vi "GetStructures.vi"(6 "error in":errorcluster, 9 "VI Interpreter in":refnum<class "VI Interpreter.lvclass">) -> (0 "error out":errorcluster, 3 "VI Interpreter out":refnum<class "VI Interpreter.lvclass">)   [LabVIEW 2014, in "VI Interpreter.lvclass"]
uses:
  VI Interpreter.lvclass
  Diagram/Diagram.lvclass/Diagram.ctl
  Structure/Structure.lvclass/Structure.ctl
  Structure/Structure.lvclass
  Diagram/Diagram.lvclass
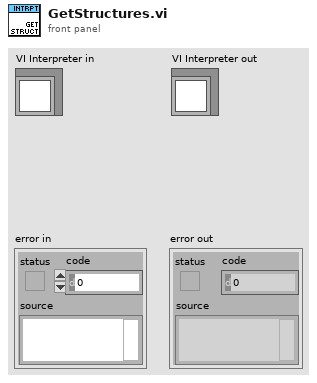
[diagram p1: front panel]
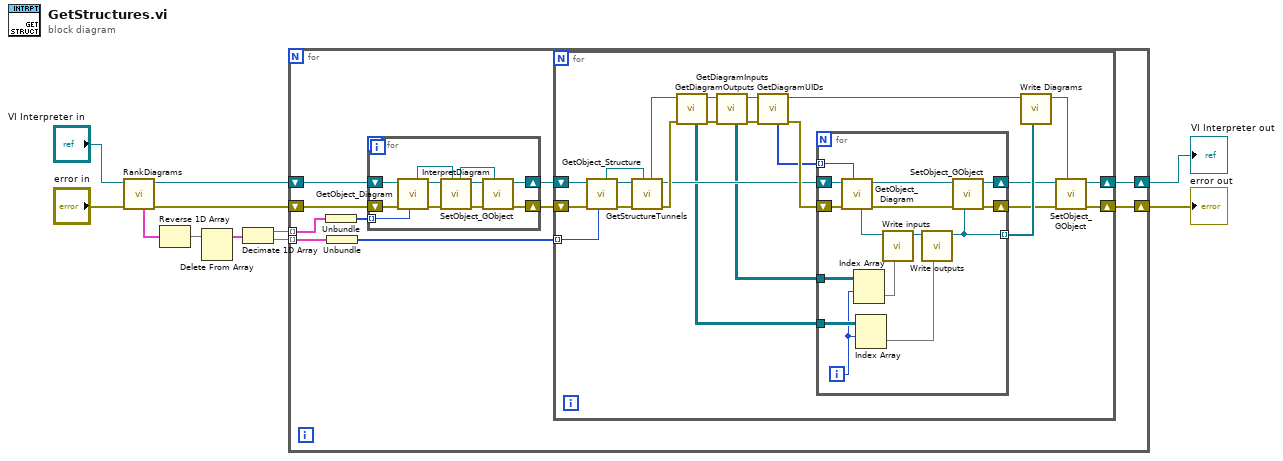
[diagram p0: block diagram]
diagram:
  n1 = call "RankDiagrams.vi"("error in"="error in", "VI Interpreter in"="VI Interpreter in") -> ("error out"=w3:errorcluster, "VI Interpreter out"=w4:refnum<class "VI Interpreter.lvclass">, "Rank"=w9:cluster{"nodes":i32[]}[])  [unwired: 5 in]
  n2 = Reverse 1D Array(array=w9) -> (reversed array=w8:cluster{"nodes":i32[]}[])
  n3 = Delete From Array(array=w8) -> (array with subset deleted=w7:cluster{"nodes":i32[]}[])  [unwired: 2 in, 1 out]
  n4 = Decimate 1D Array(w7) -> (w6:cluster{"nodes":i32[]}[], w5:cluster{"nodes":i32[]}[])
  n5 = for {
    tunnel: w6 -> [w13] mode=indexing
    tunnel: w5 -> [w21] mode=indexing
    shift-right: [w19] -> w1
    shift-left: w4 -> [w15]
    shift-right: [w18] -> w2
    shift-left: w3 -> [w17]
    n6 = Unbundle(w13) -> ("nodes"=w12:i32[])
    n7 = Unbundle(w21) -> ("nodes"=w20:i32[])
    n8 = for {
      shift-right: [w25] -> w16
      shift-left: w17 -> [w32]
      shift-right: [w26] -> w14
      shift-left: w15 -> [w31]
      tunnel: w12 -> [w22] mode=indexing
      n9 = call "GetObject_Diagram.vi"("UID"=w22, "error in"=w32, "VI Interpreter in"=w31) -> ("error out"=w29:errorcluster, "VI Interpreter out"=w30:refnum<class "VI Interpreter.lvclass">, "Diagram"=w23:refnum<class "Diagram.lvclass">)  [unwired: 3 in, 1 out]
      n10 = call "InterpretDiagram.vi"("Diagram"=w23, "error in"=w29, "VI Interpreter in"=w30) -> ("error out"=w27:errorcluster, "VI Interpreter out"=w28:refnum<class "VI Interpreter.lvclass">, "Diagram out"=w24:refnum<class "Diagram.lvclass">)  [unwired: 4 in]
      n11 = call "SetObject_GObject.vi"("GObject"=w24, "error in"=w27, "VI Interpreter in"=w28) -> ("error out"=w25:errorcluster, "VI Interpreter out"=w26:refnum<class "VI Interpreter.lvclass">)  [unwired: 5 in]
    }
    n12 = for {
      shift-right: [w35] -> w19
      shift-left: w14 -> [w56]
      tunnel: w20 -> [w54] mode=indexing
      shift-right: [w34] -> w18
      shift-left: w16 -> [w55]
      n13 = call "GetObject_Structure.vi"("UID"=w54, "error in"=w55, "VI Interpreter in"=w56) -> ("error out"=w51:errorcluster, "VI Interpreter out"=w53:refnum<class "VI Interpreter.lvclass">, "structure"=w52:refnum<class "Structure.lvclass">)  [unwired: 3 in, 1 out]
      n14 = call "GetStructureTunnels.vi"("Structure in"=w52, "error in"=w51, "VI Interpreter in"=w53) -> ("error out"=w45:errorcluster, "VI Interpreter out"=w43:refnum<class "VI Interpreter.lvclass">, "Structure out"=w48:refnum<class "Structure.lvclass">)  [unwired: 4 in]
      n15 = call-dynamic "GetDiagramOutputs.vi"("error in"=w45, "Structure in"=w48) -> ("error out"=w47:errorcluster, "Structure out"=w50:refnum<class "Structure.lvclass">, "output terminals"=w40:refnum<class "Terminal.lvclass">[][])  [unwired: 5 in]
      n16 = call-dynamic "GetDiagramInputs.vi"("error in"=w47, "Structure in"=w50) -> ("error out"=w46:errorcluster, "Structure out"=w49:refnum<class "Structure.lvclass">, "inputs terminals"=w41:refnum<class "Terminal.lvclass">[][])  [unwired: 5 in]
      n17 = call-dynamic "GetDiagramUIDs.vi"("error in"=w46, "Structure in"=w49) -> ("error out"=w44:errorcluster, "Structure out"=w39:refnum<class "Structure.lvclass">, "diagrams"=w42:i32[])  [unwired: 5 in]
      n18 = for {
        shift-right: [w64] -> w36
        shift-left: w44 -> [w71]
        shift-right: [w63] -> w37
        shift-left: w43 -> [w70]
        tunnel: w42 -> [w69] mode=indexing
        tunnel: w41 -> [w59]
        tunnel: w40 -> [w61]
        tunnel: [w62] -> w38 mode=indexing
        i -> [w57]
        n19 = call "GetObject_Diagram.vi"("UID"=w69, "error in"=w71, "VI Interpreter in"=w70) -> ("error out"=w65:errorcluster, "VI Interpreter out"=w66:refnum<class "VI Interpreter.lvclass">, "Diagram"=w68:refnum<class "Diagram.lvclass">)  [unwired: 3 in, 1 out]
        n20 = Index Array(array=w59, index (row)=w57) -> (element=w58:refnum<class "Terminal.lvclass">[])  [unwired: 1 in]
        n21 = Index Array(array=w61, index (row)=w57) -> (element=w60:refnum<class "Terminal.lvclass">[])  [unwired: 1 in]
        n22 = call "Write inputs.vi"("inputs"=w58, "Diagram in"=w68) -> ("Diagram out"=w67:refnum<class "Diagram.lvclass">)  [unwired: 7 in]
        n23 = call "Write outputs.vi"("outputs"=w60, "Diagram in"=w67) -> ("Diagram out"=w62:refnum<class "Diagram.lvclass">)  [unwired: 7 in]
        n24 = call "SetObject_GObject.vi"("GObject"=w62, "error in"=w65, "VI Interpreter in"=w66) -> ("error out"=w64:errorcluster, "VI Interpreter out"=w63:refnum<class "VI Interpreter.lvclass">)  [unwired: 5 in]
      }
      n25 = call "Write Diagrams.vi"("Diagrams"=w38, "Structure in"=w39) -> ("Structure out"=w33:refnum<class "Structure.lvclass">)  [unwired: 7 in]
      n26 = call "SetObject_GObject.vi"("GObject"=w33, "error in"=w36, "VI Interpreter in"=w37) -> ("error out"=w34:errorcluster, "VI Interpreter out"=w35:refnum<class "VI Interpreter.lvclass">)  [unwired: 5 in]
    }
  }
  "error out" <- w2
  "VI Interpreter out" <- w1
